vi "Search 1D Array.vi"(0 "JSON Value in":refnum<class "JSON Value.lvclass">, 7 "JSON Value in":refnum<class "JSON Value.lvclass">, 9 "start index (0)":i32, 11 "error in (no error)":errorcluster) -> (8 "index of element":i32, 15 "error out":errorcluster)   [LabVIEW 2016, in "JSON Value.lvclass"]
doc: "Searches for an element in a 1D array starting at start index. Because the search is linear, you need not sort the array before calling this function. LabVIEW stops searching as soon as the element is found."
uses:
  JSON Value.lvclass
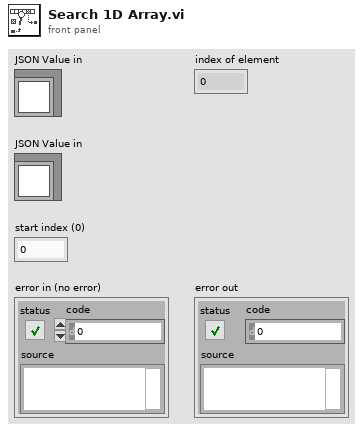
[diagram p1: front panel]
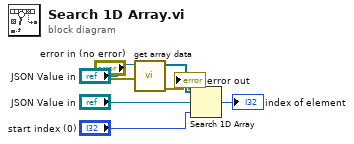
[diagram p0: block diagram]
diagram:
  n1 = call "get array data.vi"("error in (no error)"="error in (no error)", "JSON Value in"="JSON Value in") -> ("error out"=→"error out":errorcluster, "JSON Array out"=w4:refnum<class "JSON Value.lvclass">[])  [unwired: 8 in]
  n2 = Search 1D Array(1D array=w4, element="JSON Value in", start index (0)="start index (0)") -> (index of element=→"index of element":i32)
